vi "scheduleUpdate.vi"(8 "error in (no error)":errorcluster, 11 "Model in":refnum<class "Model.lvclass">) -> (0 "error out":errorcluster, 3 "Model out":refnum<class "Model.lvclass">)   [LabVIEW 2015, in "Model.lvclass"]
uses:
  Model.lvclass
  Typedefs/CommandSelector.ctl
  Model.lvclass/Model.ctl
  UserEvents/UserEvents.lvclass/UserEvents.ctl
  ICommandFactory/ICommandFactory.lvclass
  UserEvents/UserEvents.lvclass
  Typedefs/FAMTTypedefs.lvlib
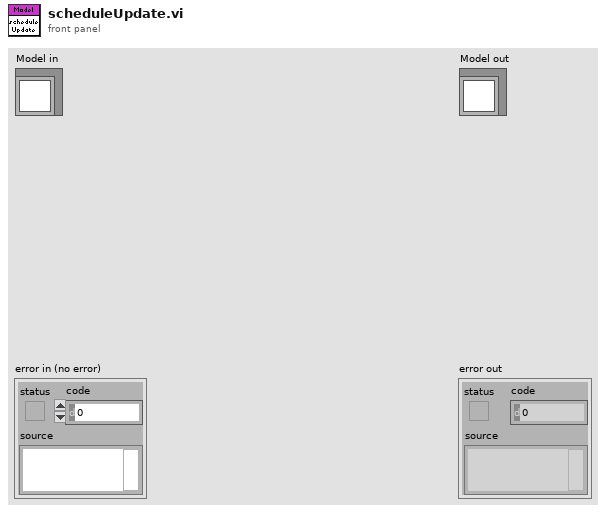
[diagram p1: front panel]
types:
  T1 = typedef "FAMTTypedefs.lvlib/CommandSelector.ctl" = enum16{"Start", "Enable", "Disable", "Standby", "Shutdown", "Update"}
  T2 = typedef "FAMTTypedefs.lvlib/SubDataEvents.ctl" = cluster{"Command":refnum<user-event>}
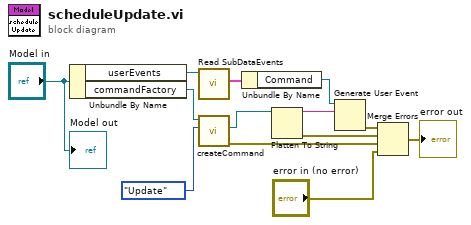
[diagram p0: block diagram]
diagram:
  n1 = Unbundle By Name("Model in") -> ("userEvents"=w12:refnum<class "UserEvents.lvclass">, "commandFactory"=w10:refnum<class "ICommandFactory.lvclass">)
  n2 = call "Read SubDataEvents.vi"("UserEvents in"=w12) -> ("SubDataEvents"=w11:T2)  [unwired: 9 in, 1 out]
  n3 = call-dynamic "createCommand.vi"("Command"=CommandSelector."Update", "ICommandFactory in"=w10) -> ("error out"=w4:errorcluster, "command"=w8:refnum<class "Command.lvclass">)  [unwired: 7 in, 1 out]
  n4 = Unbundle By Name(w11) -> ("Command"=w6:refnum<user-event>)
  n5 = Flatten To String(anything=w8) -> (data string=w7:string, error out=w3:errorcluster)  [unwired: 3 in, 1 out]
  n6 = Generate User Event(user event=w6, event data cluster=w7) -> (error out=w2:errorcluster)  [unwired: 2 in, 1 out]
  n7 = Merge Errors(w2, w3, w4, "error in (no error)") -> (→"error out":errorcluster)
  "Model out" <- "Model in"
